vi "ap free handle.vi"(11 "ap_handle":u32) -> (2 "function return":i32, 3 "ap_handle out":u32)   [LabVIEW 2019, in "apdm.lvlib"]
doc: "APDM_EXPORT int apdm_ap_free_handle(apdm_ap_handle_t ap_handle);"
uses:
  apdm.lvlib
  Lee Lab/CP FES Walking 2018/Code/Working/LabVIEW/apdm.dll
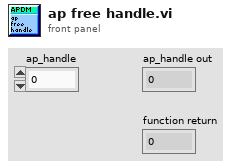
[diagram p1: front panel]
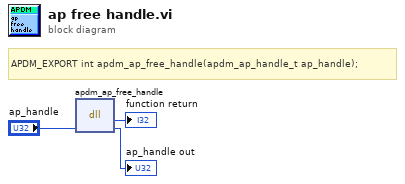
[diagram p0: block diagram]
diagram:
  # "APDM_EXPORT int apdm_ap_free_handle(apdm_ap_handle_t ap_handle);"
  n1 = dll-call lib="C:/Users/jfalesi/Dropbox/Lee Lab/CP FES Walking 2018/Code/Working/LabVIEW/apdm.*" fn="apdm_ap_free_handle"("ap_handle"="ap_handle") -> (→"function return":i32, "ap_handle"=→"ap_handle out":u32)  [unwired: 3 in, 2 out]
